vi "Write Steps to File.vi"(8 "error in (no error)":errorcluster, 11 "Macro in":refnum<class "Macro.lvclass">) -> (0 "error out":errorcluster, 3 "Macro out":refnum<class "Macro.lvclass">)   [LabVIEW 2020, in "MacroAssert.lvlib" / "Macro.lvclass"]
uses:
  Macro.lvclass
  Macro.lvclass/Macro.ctl
  Step/Step.lvclass
  MacroAssert.lvlib
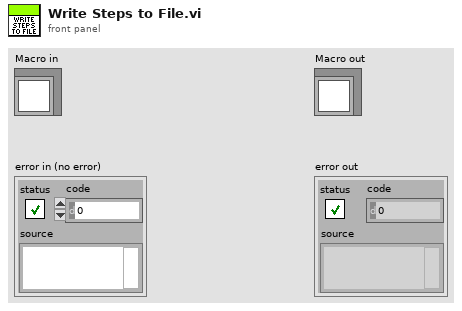
[diagram p1: front panel]
types:
  T1 = typedef "NI_LVConfig.lvlib/Config Data RefNum.ctl" = refnum<k1>
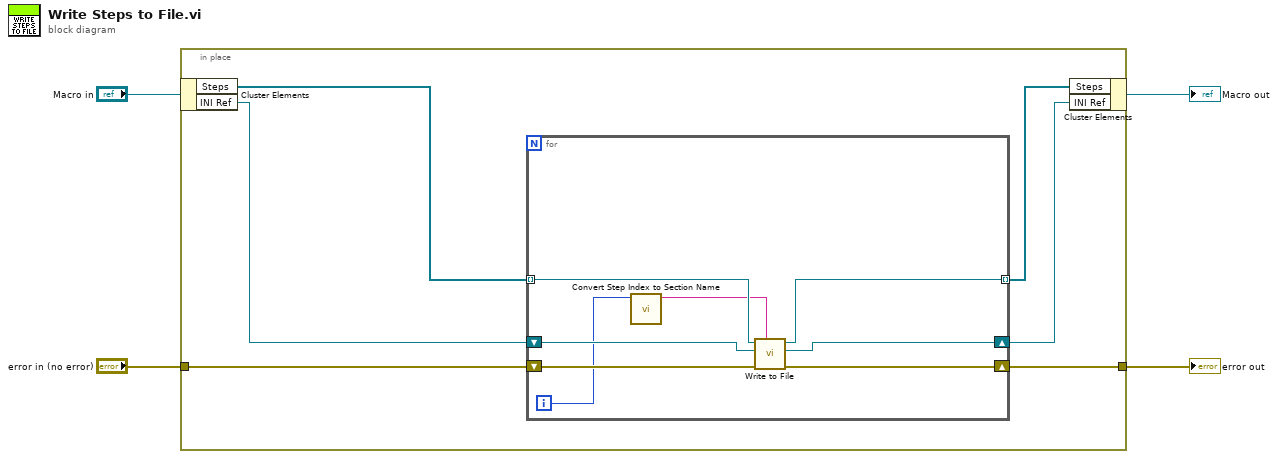
[diagram p0: block diagram]
diagram:
  n1 = in-place {
    in-place-border: "error in (no error)" -> [w8]
    in-place-border: [w10] -> w1
    n2 = in-place-cluster #1("Macro in") -> ("Steps"=w6:refnum<class "Step.lvclass">[], "INI Ref"=w7:T1)
    n3 = for {
      shift-right: [w17] -> w10
      shift-left: w8 -> [w15]
      shift-right: [w16] -> w9
      shift-left: w7 -> [w18]
      tunnel: w6 -> [w14] mode=indexing
      tunnel: [w13] -> w5 mode=indexing
      i -> [w12]
      n4 = call "Convert Step Index to Section Name.vi"("Step Index"=w12) -> ("Section Name"=w11:string)  [unwired: 10 in]
      n5 = call-dynamic "Write to File.vi"("Section Name"=w11, "error in (no error)"=w15, "INI Ref"=w18, "Step in"=w14) -> ("error out"=w17:errorcluster, "INI Ref out"=w16:T1, "Step out"=w13:refnum<class "Step.lvclass">)  [unwired: 5 in]
    }
    n6 = in-place-cluster #1("Steps"=w5, "INI Ref"=w9) -> (→"Macro out":refnum<class "Macro.lvclass">)
  }
  "error out" <- w1
